vi "Minutes to Start Time.vi"(8 "error in (no error)":errorcluster, 11 "Minutes":i32) -> (0 "error out":errorcluster, 3 "Simulated Time":string)   [LabVIEW 2026]
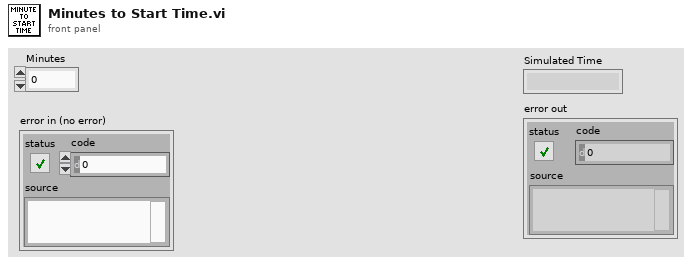
[diagram p1: front panel]
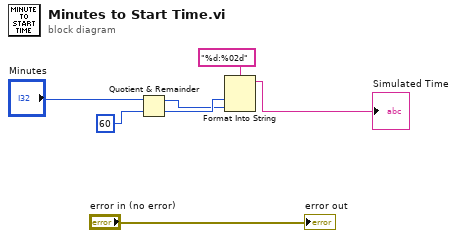
[diagram p0: block diagram]
diagram:
  n1 = Quotient & Remainder(x="Minutes", y=60) -> (x-y*floor(x/y)=w2:i32, floor(x/y)=w3:i32)
  n2 = Format Into String(format string="%d:%02d", w3, w2) -> (resulting string=→"Simulated Time":string)  [unwired: 2 in, 1 out]
  "error out" <- "error in (no error)"
